vi "GearFlap.vi"(11 "Gear Flap":bool) -> ()   [LabVIEW 2017]
uses:
  <vilib>/Rock Robotics/WPI/Solenoid/Deprecated/WPI_SolenoidSetBool.vi
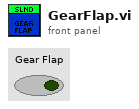
[diagram p1: front panel]
types:
  T1 = typedef "WPI_SolenoidDevRef.ctl" = cluster{"DevStatus":errorcluster, "Pneumatics Control Module":u8, "Forward Solenoid Channel":T2, "Reverse Solenoid Channel":T2}
  T2 = typedef "WPI_SolenoidChannel.ctl" = enum8{"Solenoid 0", "Solenoid 1", "Solenoid 2", "Solenoid 3", "Solenoid 4", "Solenoid 5", "Solenoid 6", "Solenoid 7", "Invalid"}
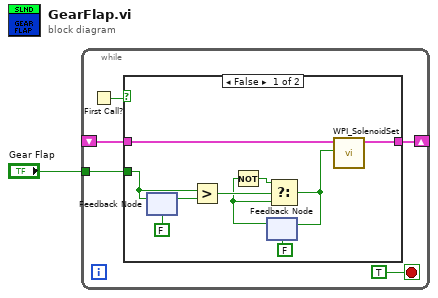
[diagram p0: block diagram]
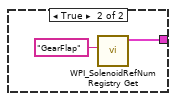
[diagram p2: hidden frame]
diagram:
  n1 = while {
    tunnel: "Gear Flap" -> [w5]
    shift-right: [w4] -> _
    shift-left: _ -> [w3]
    stop <- TRUE stop-if-true
    n2 = First Call?() -> (First Call?: T/F=w2:bool)
    n3 = case shown="False" w2 {
      tunnel: w5 -> [w9 _]
      tunnel: [w16 w18] -> w4
      tunnel: w3 -> [w7 _]
      frame False {
        n4 = feedback #1(FALSE ("Fuel Flap")) -> (w14:bool)
        n5 = feedback-in #1(w9) -> ()
        n6 = Greater?(x=w9, y=w14) -> (0:w13:bool)
        n7 = feedback #2(FALSE) -> (w11:bool)
        n8 = Not(x=w11) -> (.not. x?=w12:bool)
        n9 = Select(t=w12, s=w13, f=w11) -> (s? t:f=w8:bool)
        n10 = feedback-in #2(w8) -> ()
        n11 = call-poly <vilib>:"WPI_SolenoidSet.vi"("Value"=w8, "SolenoidDevRef"=w7) -> ("SolenoidDevRef"=w16:T1)  [unwired: 8 in, 1 out]
      }
      frame True {
        n12 = call <vilib>:"WPI_SolenoidRefNum Registry Get.vi"("refnum name"="GearFlap") -> ("SolenoidDevRef"=w18:T1)  [unwired: 9 in, 1 out]
      }
    }
  }
